vi "Subvi buffer test.vi"(0 "Cluster in":cluster{"FIFO name":refnum<k21>, "timeout":i32}={"FIFO name"="FIFO", "timeout"=0}) -> ()   [LabVIEW 2017]
uses:
  <vilib>/rvi/DataTransferAndStorage/Container/Common/niFpgaContainerExecOnDevCompGetState.vi
  <vilib>/rvi/Emulation/niFpgaEmulationIsFPGAContextNoSignature.vi
  <vilib>/rvi/Emulation/niFpgaSctlEmulationGetInTimedLoop.vi
  <vilib>/rvi/errors/niFpgaSetErrorForExecOnDevCompSimple.vi
  <vilib>/rvi/eio/common/nirviEmuReportErrorAndStop.vi
  <vilib>/rvi/DataTransferAndStorage/Container/Common/niFpgaContainerGetUniqueNameForEmu.vi
  <vilib>/rvi/FIFO/Fifo_Resource/nirvififoEmulationSetSize.vi
  <vilib>/rvi/FIFO/Fifo_Resource/nirviFifoEmulationQueueMgr.vi
  <instcachedir>/0/nirviFifoEmulationQueueMgr_E5CAEC123FF24DC58D834DCA3CDAA9B5.lvgen/nirviFifoEmulationQueueMgr_E5CAEC123FF24DC58D834DCA3CDAA9B5_001.vi
  <vilib>/rvi/FIFO/Fifo_Resource/nirvififoEmulationDetermineInputValidOut.vi
  <vilib>/rvi/FIFO/Fifo_Resource/nirvififoEmulationCreateLock.vi
  <vilib>/rvi/Emulation/niFpgaProcessEmulError.vi
  <vilib>/rvi/FIFO/Fifo_Resource/nirvififoEmulationObtainLock.vi
  <vilib>/rvi/FIFO/Fifo_Resource/nirvififoEmulationReleaseLock.vi
  <vilib>/rvi/occurrence/nirviWaitOnOccurrenceBase.vi
  <vilib>/rvi/errors/nirviReportUnexpectedCaseInternalError.vi
  <vilib>/rvi/errors/nirviReportUnexpectedCaseInternalError (U32).vi
  <vilib>/Utility/error.llb/Clear Errors.vi
  <vilib>/rvi/interface/RandomDataEmulation/niFpgaRandomDataHandleErrors.vi
  <vilib>/rvi/DataTransferAndStorage/Container/XNode/niFpgaContainer.xnode
  <vilib>/rvi/FIFO/Fifo_Resource/niFpgaFifoEmulationRefIn.vi
  <vilib>/rvi/FIFO/Fifo_Resource/nirvififoEmulationWrite.vi
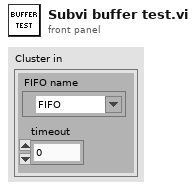
[diagram p1: front panel]
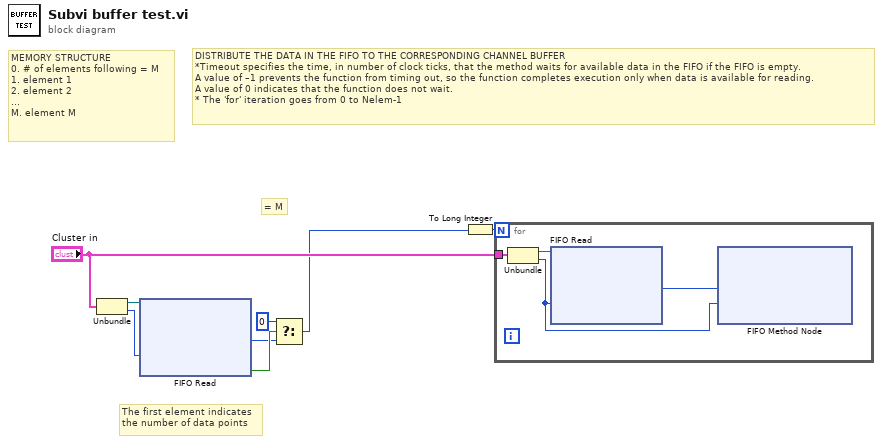
[diagram p0: block diagram]
diagram:
  # "= M"
  # "MEMORY STRUCTURE\n0. # of elements following = M\n1. element 1\n2. element 2\n...\nM. element M"
  # "The first element indicates\nthe number of data points"
  # "DISTRIBUTE THE DATA IN THE FIFO TO THE CORRESPONDING CHANNEL BUFFER\n*Timeout specifies the time, in number of clock ticks, that the method waits for available data in the FIFO if the FIFO is empty.\nA value of –1 prevents the function from timing out, so the function completes execution only when data is available for reading.\nA value of 0 indicates that the function does not wait.\n* The 'for' iteration goes from 0 to Nelem-1"
  n1 = Unbundle("Cluster in") -> ("FIFO name"=w8:refnum<k21>, "timeout"=w1:i32)
  n2 = xnode ("FIFO Read")("Timeout"=w1, "FIFO In"=w8) -> ("Element"=w6:u32, "Timed Out?"=w7:bool)  [unwired: 1 out]
  n3 = Select(t=u32 0, s=w7, f=w6) -> (s? t:f=w2:u32)
  n4 = To Long Integer(number=w2) -> (32bit integer=w3:i32)
  n5 = for {
    N: w3 -> [_]
    tunnel: "Cluster in" -> [w12]
    n6 = Unbundle(w12) -> ("FIFO name"=w11:refnum<k21>, "timeout"=w9:i32)
    n7 = xnode ("FIFO Read")("FIFO In"=w11, "Timeout"=w9) -> ("Element"=w10:u32)  [unwired: 2 out]
    n8 = xnode ("FIFO Method Node")("Element"=w10, "Timeout"=w9) -> ()  [unwired: 1 in, 2 out]
  }
